vi "PatchSystemDefinitionFile.vi"(7 "VI in":refnum<vi>, 8 "error in (no error)":errorcluster, 9 "overrides files":path[](array[path]), 10 "System Definition File":path, 11 "VeriStand Test Case in":refnum<class "VeriStandTestCase.lvclass">) -> (0 "error out":errorcluster, 2 "absolute overridden system definition file":path, 3 "VeriStand Test Case out":refnum<class "VeriStandTestCase.lvclass">)   [LabVIEW 2016, in "VeriStandTestCase.lvclass"]
uses:
  VeriStandTestCase.lvclass
  VeriStandTestCase.lvclass/VeriStandTestCase.ctl
  VeriStandTestUtilities/VeriStandTestUtilities.lvlib
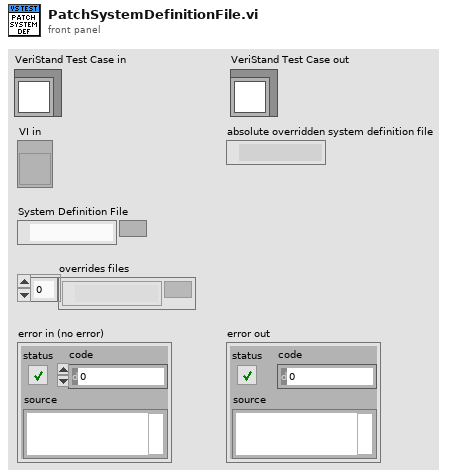
[diagram p1: front panel]
types:
  T1 = typedef "VeriStandTestUtilities.lvlib/ConfigPropertyItem.ctl" = cluster{"key":string, "value":string}
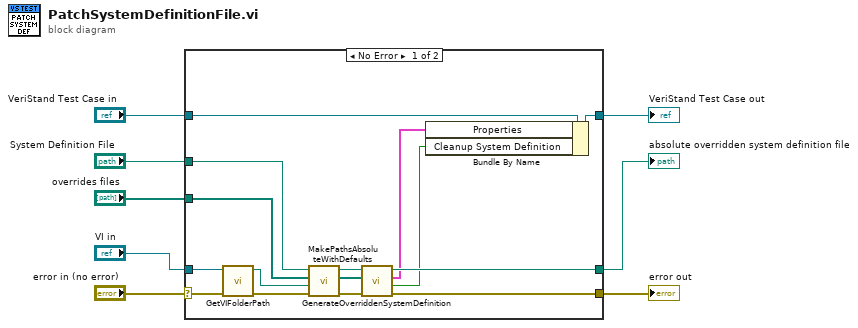
[diagram p0: block diagram]
diagram:
  n1 = case shown="No Error" "error in (no error)" {
    selector: "error in (no error)" -> [w13 w25]
    tunnel: "VI in" -> [w22 _]
    tunnel: [w20 _] -> w7
    tunnel: [w19 w25] -> w6
    tunnel: "System Definition File" -> [w15 _]
    tunnel: "overrides files" -> [w14 _]
    tunnel: "VeriStand Test Case in" -> [w12 w24]
    tunnel: [w11 w24] -> w1
    frame No Error {
      n2 = call "GetVIFolderPath.vi"("error in (no error)"=w13, "VI Reference in"=w22) -> ("error out"=w21:errorcluster, "VI Folder Path out"=w23:path)  [unwired: 8 in]
      n3 = call "MakePathsAbsoluteWithDefaults.vi"("error in (no error)"=w21, "relative base path"=w23, "overrides files"=w14, "system definition file"=w15) -> ("error out"=w18:errorcluster, "absolute overrides files"=w17:path[], "absolute system definition file"=w16:path)  [unwired: 5 in]
      n4 = call "GenerateOverriddenSystemDefinition.vi"("error in (no error)"=w18, "absolute configuration files"=w17, "absolute system definition file"=w16) -> ("error out"=w19:errorcluster, "Temporary File?"=w9:bool, "properties"=w10:T1[], "absolute overridden system definition file"=w20:path)  [unwired: 5 in]
      n5 = Bundle By Name(cluster=w12, "Properties"=w10, "Cleanup System Definition"=w9) -> (w11:refnum<class "VeriStandTestCase.lvclass">)
    }
    frame Error {
    }
  }
  "absolute overridden system definition file" <- w7
  "error out" <- w6
  "VeriStand Test Case out" <- w1
